vi "Stop Core.vi"(10 "final error code":i32, 11 "ePAS in":refnum<class "ePAS.lvclass">) -> (3 "ePAS out":refnum<class "ePAS.lvclass">)   [LabVIEW 2014, in "PAS Actor Lib.lvlib" / "ePAS.lvclass"]
doc: "(<B>Filename</B>: Actor Framework.lvlib:Actor.lvclass:Stop Core.vi)\n\nDefines what the actor does before it stops. Use the <B>final error code</B> input to determine whether the actor shut down in response to an error.\n\nBy default, this method does nothing. A descendant class may override it to define behavior, such as shutting down any processes the actor initiated in its override of the Actor Core method."
uses:
  ePAS.lvclass
  Instr Actor/Instr Actor.lvclass
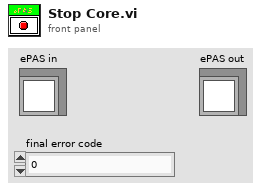
[diagram p1: front panel]
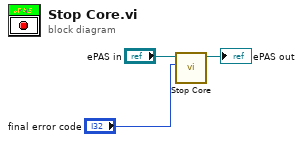
[diagram p0: block diagram]
diagram:
  n1 = call-parent "Stop Core.vi"("final error code"="final error code", "Instr Actor in"="ePAS in") -> ("Instr Actor out"=→"ePAS out":refnum<class "ePAS.lvclass">)  [unwired: 9 in]
